vi "FPGA_RC-filter.vi"(7 "deltaT/tau":fxp<+,25,0>, 9 "X_n":fxp<+/-,32,5>, 10 "mesure":fxp<+/-,26,5>) -> (2 "X_n+1":fxp<+/-,32,5> format="%.54g")   [LabVIEW 2010]
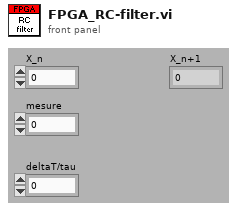
[diagram p1: front panel]
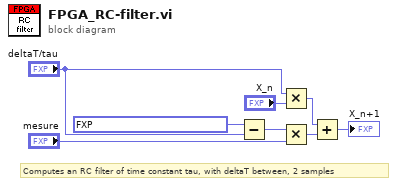
[diagram p0: block diagram]
diagram:
  # "Computes an RC filter of time constant tau, with deltaT between, 2 samples"
  n1 = Subtract(x=fxp<+/-,26,5> 1.0, y="deltaT/tau") -> (x-y=w4:fxp<+/-,31,6>)
  n2 = Multiply(x="deltaT/tau", y="X_n") -> (x*y=w2:fxp<+/-,57,5>)
  n3 = Multiply(x=w4, y="mesure") -> (x*y=w3:fxp<+/-,52,5>)
  n4 = Add(x=w2, y=w3) -> (x+y=→"X_n+1":fxp<+/-,32,5>)
